vi "hex合法检测.vi"(1 "字符串输入":string) -> (0 "x与y？":bool)   [LabVIEW 2016]
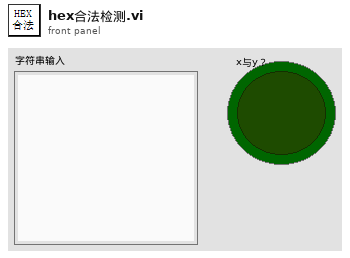
[diagram p1: front panel]
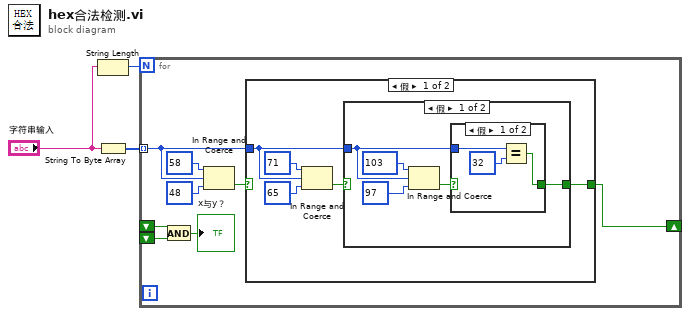
[diagram p0: block diagram]
diagram:
  n1 = String Length(string="字符串输入") -> (length=w3:i32)
  n2 = String To Byte Array(string="字符串输入") -> (unsigned byte array=w1:u8[])
  n3 = for {
    N: w3 -> [_]
    tunnel: w1 -> [w8] mode=indexing
    shift-right: [w7] -> _
    shift-left: _ -> [w6]
    shift-left: _ -> [w5]
    n4 = And(x=w6, y=w5) -> (x .and. y?=→"x与y？":bool)
    n5 = In Range and Coerce(upper limit=u8 58 ("上限"), x=w8, lower limit=u8 48 ("下限")) -> (In Range?=w9:bool)  [unwired: 1 out]
    n6 = case shown="假" w9 {
      selector: w9 -> [_ w27]
      tunnel: w8 -> [w13 _]
      tunnel: [w12 w27] -> w7
      frame False {
        n7 = In Range and Coerce(upper limit=u8 71 ("上限"), x=w13, lower limit=u8 65 ("下限")) -> (In Range?=w14:bool)  [unwired: 1 out]
        n8 = case shown="假" w14 {
          selector: w14 -> [_ w26]
          tunnel: w13 -> [w17 _]
          tunnel: [w18 w26] -> w12
          frame False {
            n9 = In Range and Coerce(upper limit=u8 103 ("上限"), x=w17, lower limit=u8 97 ("下限")) -> (In Range?=w19:bool)  [unwired: 1 out]
            n10 = case shown="假" w19 {
              selector: w19 -> [_ w25]
              tunnel: [w22 w25] -> w18
              tunnel: w17 -> [w24 _]
              frame False {
                n11 = Equal?(x=w24, y=u8 32) -> (x = y?=w22:bool)
              }
              frame True {
              }
            }
          }
          frame True {
          }
        }
      }
      frame True {
      }
    }
  }
